vi "FT10_Semi-Auto 2 Tester.vi"(7 "Read/ Write":T10, 8 "Error In":errorcluster, 10 "Semi-Auto 2 Cluster in":T1, 11 "Path":path=path "C:/Users/yearon2/OneDrive - Medtronic PLC/LV2024/LT10 Generator Sandbox/FT10_rev2/Semi-Auto 2 Commands.csv") -> (0 "Error Out":errorcluster, 2 "Semi-Auto 2 Cluster out":T1, 3 "Semi-Auto 2-D Array out":T9)   [LabVIEW 2024]
uses:
  NI Online Practice/CLD Practice/cld_success_package/Preparation_Materials/CLD 6/CLD 6 CSV file enum.ctl
  Controls/Control_Semi-Auto 2-D Array.ctl
  Controls/Control_Semi-Auto Cluster Array 2.ctl
  Controls/Control_Semi-Auto Cluster 2.ctl
  Controls/Control_Semi-Auto Mode.ctl
  Controls/Control_Semi-Auto Unitherm Load.ctl
  Controls/Control_Semi-Auto Power Level.ctl
  Controls/Control_Semi-Auto Activation Duration.ctl
  Controls/Control_Semi-Auto Port.ctl
  Controls/Control_Semi-Auto 2 Activation Method.ctl
  Controls/Control_Semi-Auto 1-D Array.ctl
  <vilib>/Utility/file.llb/Read Delimited Spreadsheet (string).vi
  <vilib>/Utility/file.llb/Write Delimited Spreadsheet (string).vi
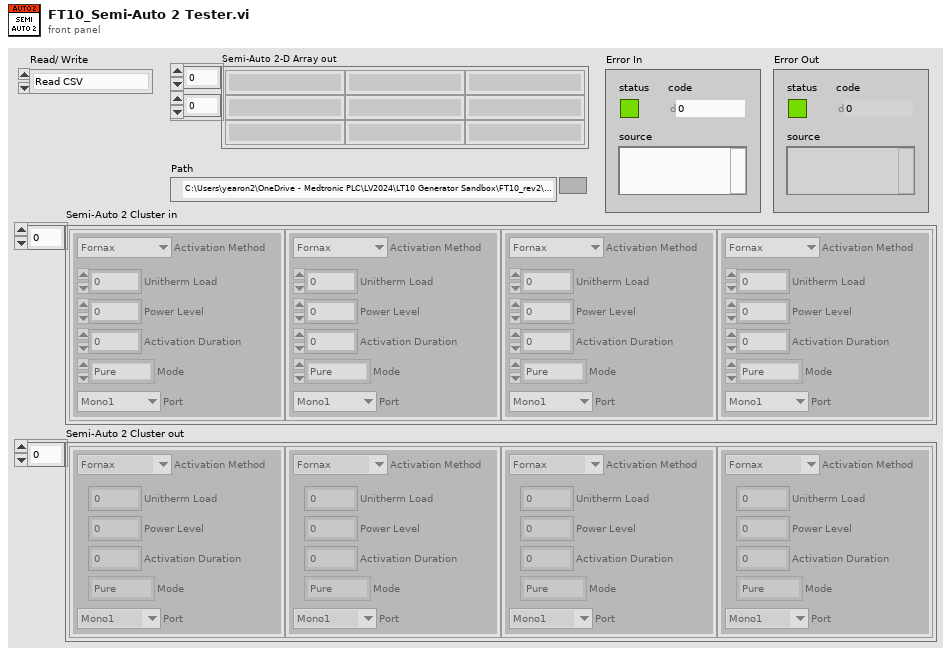
[diagram p1: front panel]
types:
  T1 = typedef "Control_Semi-Auto Cluster Array 2.ctl" = T2[]
  T2 = typedef "Control_Semi-Auto Cluster 2.ctl" = cluster{"Mode":T3, "Unitherm Load":T4, "Power Level":T5, "Activation Duration":T6, "Port":T7, "Activation Method":T8}
  T3 = typedef "Control_Semi-Auto Mode.ctl" = enum16{"Pure", "Blend", "Spray", "Fulgerate", "Standard", "Macro", "Precision", "Ligasure", "Error"}
  T4 = typedef "Control_Semi-Auto Unitherm Load.ctl" = i32
  T5 = typedef "Control_Semi-Auto Power Level.ctl" = dbl
  T6 = typedef "Control_Semi-Auto Activation Duration.ctl" = i32
  T7 = typedef "Control_Semi-Auto Port.ctl" = enum16{"Mono1", "Mono2", "Bipolar", "Ligasure", "Error"}
  T8 = typedef "Control_Semi-Auto 2 Activation Method.ctl" = enum16{"Fornax", "Handswitch", "Footswitch"}
  T9 = typedef "Control_Semi-Auto 2-D Array.ctl" = string[][]
  T10 = typedef "CLD 6 CSV file enum.ctl" = enum16{"Read CSV", "Write CSV"}
  T11 = typedef "Control_Semi-Auto 1-D Array.ctl" = string[]
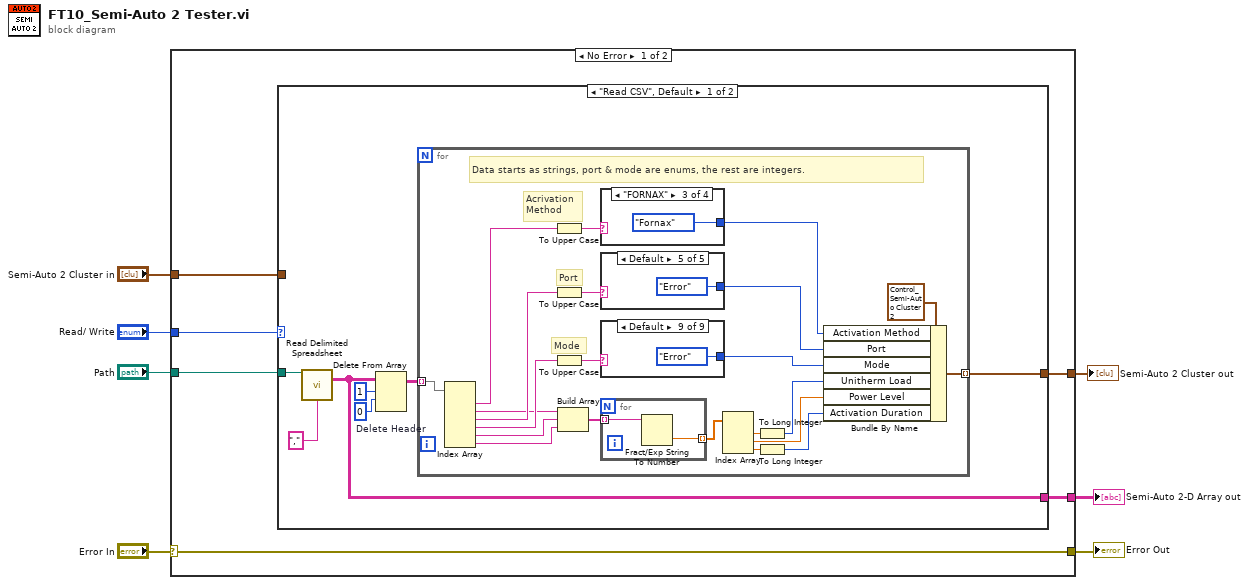
[diagram p0: block diagram]
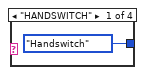
[diagram p2: hidden frame]
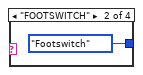
[diagram p3: hidden frame]
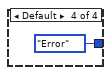
[diagram p4: hidden frame]
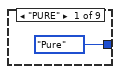
[diagram p5: hidden frame]
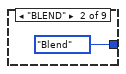
[diagram p6: hidden frame]
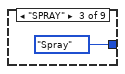
[diagram p7: hidden frame]
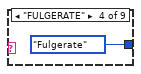
[diagram p8: hidden frame]
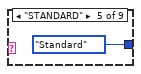
[diagram p9: hidden frame]
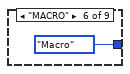
[diagram p10: hidden frame]
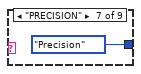
[diagram p11: hidden frame]
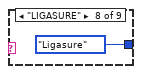
[diagram p12: hidden frame]
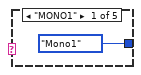
[diagram p13: hidden frame]
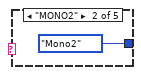
[diagram p14: hidden frame]
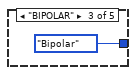
[diagram p15: hidden frame]
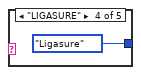
[diagram p16: hidden frame]
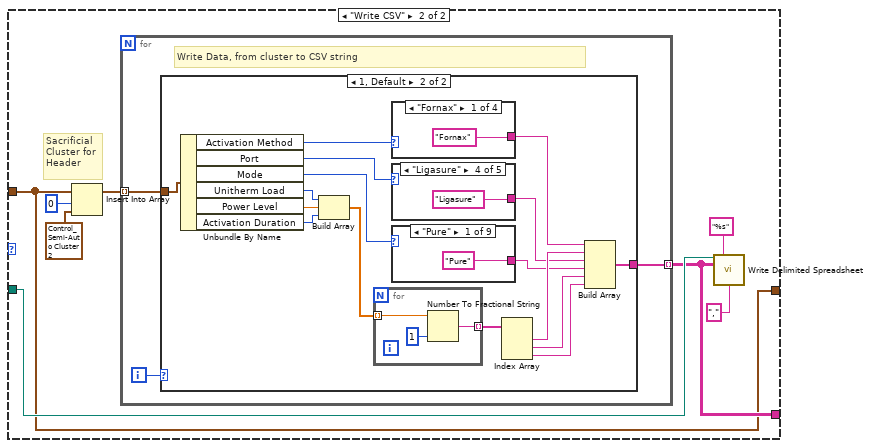
[diagram p17: hidden frame]
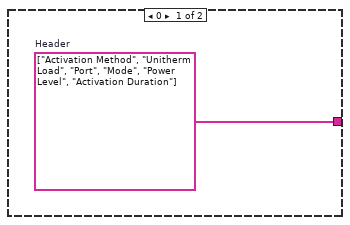
[diagram p18: hidden frame]
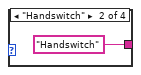
[diagram p19: hidden frame]
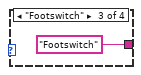
[diagram p20: hidden frame]
diagram:
  n1 = case shown="No Error" "Error In" {
    selector: "Error In" -> [w10 w114]
    tunnel: [w13 T1 [] ("Semi-Auto 2 Cluster in")] -> w1
    tunnel: "Path" -> [w8 _]
    tunnel: "Read/ Write" -> [w12 _]
    tunnel: "Semi-Auto 2 Cluster in" -> [w11 _]
    tunnel: [w10 w114] -> w4
    tunnel: [w9 string[][] [] ("all rows")] -> w3
    frame No Error {
      n2 = case shown="\"Read CSV\", Default" w12 {
        tunnel: w8 -> [w19 w69]
        tunnel: [w20 w66] -> w13
        tunnel: w11 -> [_ w66]
        tunnel: [w17 w67] -> w9
        frame "Read CSV", Default {
          n3 = call-poly <vilib>:"Read Delimited Spreadsheet.vi"("file path (dialog if empty)"=w19, "delimiter (\\t)"="," ("delimiter (\\t)")) -> ("all rows"=w17:string[][])  [unwired: 8 in, 5 out]
          n4 = Delete From Array "Delete Header"(array=w17, length=1, index (row)=0) -> (array with subset deleted=w16:string[][])  [unwired: 1 in, 1 out]
          n5 = for {
            tunnel: w16 -> [w42] mode=indexing
            tunnel: [w30] -> w20 mode=indexing
            # "Acrivation \nMethod"
            # "Mode"
            # "Port"
            # "Data starts as strings, port & mode are enums, the rest are integers."
            n6 = Index Array "Index Array"(array=w42) -> (element #1=w23:string, element #2=w24:string, element #3=w25:string, element #4=w26:string, element #5=w27:string, element #6=w28:string)  [unwired: 6 in]
            n7 = To Upper Case(1:w23) -> (0:w22:string)
            n8 = To Upper Case(1:w25) -> (0:w37:string)
            n9 = To Upper Case(1:w26) -> (0:w38:string)
            n10 = Build Array(w24, w27, w28) -> (w41:string[])
            n11 = case shown="\"FORNAX\"" w22 {
              tunnel: [enum16{"Fornax", "Handswitch", "Footswitch"}."Handswitch" ("Activation Method") enum16{"Fornax", "Handswitch", "Footswitch"}."Footswitch" ("Activation Method") enum16{"Fornax", "Handswitch", "Footswitch"}."Fornax" ("Activation Method") Control_Semi-Auto_Port."Error" ("Port")] -> w21
              frame "HANDSWITCH" {
              }
              frame "FOOTSWITCH" {
              }
              frame "FORNAX" {
              }
              frame Default {
              }
            }
            n12 = case shown="Default" w37 {
              tunnel: [Control_Semi-Auto_Port."Mono1" ("Port") Control_Semi-Auto_Port."Mono2" ("Port") Control_Semi-Auto_Port."Bipolar" ("Port") Control_Semi-Auto_Port."Ligasure" ("Port") Control_Semi-Auto_Port."Error" ("Port")] -> w36
              frame "MONO1" {
              }
              frame "MONO2" {
              }
              frame "BIPOLAR" {
              }
              frame "LIGASURE" {
              }
              frame Default {
              }
            }
            n13 = case shown="Default" w38 {
              tunnel: [Control_Semi-Auto_Mode."Pure" ("Mode") Control_Semi-Auto_Mode."Blend" ("Mode") Control_Semi-Auto_Mode."Spray" ("Mode") Control_Semi-Auto_Mode."Fulgerate" ("Mode") Control_Semi-Auto_Mode."Standard" ("Mode") Control_Semi-Auto_Mode."Macro" ("Mode") Control_Semi-Auto_Mode."Precision" ("Mode") Control_Semi-Auto_Mode."Ligasure" ("Mode") Control_Semi-Auto_Mode."Error" ("Mode")] -> w35
              frame "PURE" {
              }
              frame "BLEND" {
              }
              frame "SPRAY" {
              }
              frame "FULGERATE" {
              }
              frame "STANDARD" {
              }
              frame "MACRO" {
              }
              frame "PRECISION" {
              }
              frame "LIGASURE" {
              }
              frame Default {
              }
            }
            n14 = for {
              tunnel: w41 -> [w62] mode=indexing
              tunnel: [w61] -> w40 mode=indexing
              n15 = Fract/Exp String To Number(string=w62) -> (number=w61:dbl)  [unwired: 3 in, 1 out]
            }
            n16 = Index Array "Index Array"(array=w40) -> (element #1=w33:dbl, element #2=w34:dbl, element #3=w39:dbl)  [unwired: 3 in]
            n17 = To Long Integer(number=w33) -> (32bit integer=w32:i32)
            n18 = To Long Integer(number=w39) -> (32bit integer=w31:i32)
            n19 = Bundle By Name(cluster=T2 {"Mode"=enum."Pure", "Unitherm Load"=0, "Power Level"=0.0, "Activation Duration"=0, "Port"=enum."Mono1", "Activation Method"=enum."Fornax"} ("Semi-Auto 2 Cluster in"), "Activation Method"=w21, "Port"=w36, "Mode"=w35, "Unitherm Load"=w32, "Power Level"=w34, "Activation Duration"=w31) -> (w30:T2)
          }
        }
        frame "Write CSV" {
          # "Sacrificial\nCluster for\nHeader"
          n20 = Insert Into Array(array=w66, index=0, new element=T2 {"Mode"=enum."Pure", "Unitherm Load"=0, "Power Level"=0.0, "Activation Duration"=0, "Port"=enum."Mono1", "Activation Method"=enum."Fornax"} ("Semi-Auto 2 Cluster in")) -> (w64:T1)
          n21 = for {
            tunnel: w64 -> [w73] mode=indexing
            tunnel: [w72] -> w67 mode=indexing
            i -> [w71]
            # "Write Data, from cluster to CSV string"
            n22 = case shown="1, Default" w71 {
              tunnel: w73 -> [_ w90]
              tunnel: [w74 w81] -> w72
              frame 0 {
                w74 = T11 ["Activation Method", "Unitherm Load", "Port", "Mode", "Power Level", "Activation Duration"]  # Header
              }
              frame 1, Default {
                n23 = Unbundle By Name(w90) -> ("Activation Method"=w76:T8, "Port"=w80:T7, "Mode"=w79:T3, "Unitherm Load"=w87:T4, "Power Level"=w88:T5, "Activation Duration"=w89:T6)
                n24 = Build Array(w87, w88, w89) -> (w86:T5[])
                n25 = for {
                  tunnel: w86 -> [w110] mode=indexing
                  tunnel: [w109] -> w85 mode=indexing
                  n26 = Number To Fractional String(number=w110, precision (6)=i16 1) -> (F-format string=w109:string)  [unwired: 2 in]
                }
                n27 = case shown="\"Fornax\"" w76 {
                  tunnel: ["Fornax" "Handswitch" "Footswitch" "Error"] -> w75
                  frame "Fornax" {
                  }
                  frame "Handswitch" {
                  }
                  frame "Footswitch" {
                  }
                  frame Default {
                  }
                }
                n28 = case shown="\"Ligasure\"" w80 {
                  tunnel: ["Mono1" "Mono2" "Bipolar" "Ligasure" "Error"] -> w77
                  frame "Mono1" {
                  }
                  frame "Mono2" {
                  }
                  frame "Bipolar" {
                  }
                  frame "Ligasure" {
                  }
                  frame Default {
                  }
                }
                n29 = case shown="\"Pure\"" w79 {
                  tunnel: ["Pure" "Blend" "Spray" "Fulgerate" "Standard" "Macro" "Precision" "Ligasure" "Error"] -> w78
                  frame "Pure" {
                  }
                  frame "Blend" {
                  }
                  frame "Spray" {
                  }
                  frame "Fulgerate" {
                  }
                  frame "Standard" {
                  }
                  frame "Macro" {
                  }
                  frame "Precision" {
                  }
                  frame "Ligasure" {
                  }
                  frame Default {
                  }
                }
                n30 = Index Array(array=w85) -> (element #1=w84:string, element #2=w83:string, element #3=w82:string)  [unwired: 3 in]
                n31 = Build Array(w75, w84, w77, w78, w83, w82) -> (w81:string[])
              }
            }
          }
          n32 = call-poly <vilib>:"Write Delimited Spreadsheet.vi"("file path (dialog if empty)"=w69, "format (%s)"="%s", "2D data"=w67, "delimiter (\\t)"="," ("delimiter (\\t)")) -> ()  [unwired: 10 in, 2 out]
        }
      }
    }
    frame Error {
    }
  }
  "Error Out" <- w4
  "Semi-Auto 2-D Array out" <- w3
  "Semi-Auto 2 Cluster out" <- w1
